vi "RegisterCommandPointer.vi"(10 "Strict-Typed VI Refnum":refnum<vi>, 11 "Name":string) -> ()   [LabVIEW 2011]
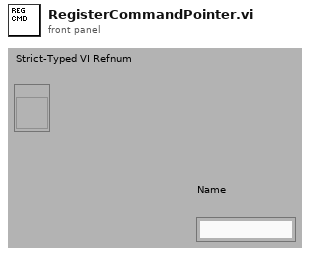
[diagram p1: front panel]
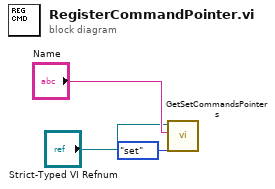
[diagram p0: block diagram]
diagram:
  n1 = call "GetSetCommandsPointers.vi"("menu"=enum16{"set", "get", "delete"}."set", "refnum name"="Name", "VI Refnum In"="Strict-Typed VI Refnum") -> ()  [unwired: 1 in, 8 out]
